vi "testSensorIdToName.vi"(8 "error in (no error)":errorcluster) -> (0 "error out":errorcluster)   [LabVIEW 2016]
doc: "Test the to map the sensor Id to sensor abbreviated name."
uses:
  <vilib>/addons/_JKI Toolkits/Caraya/classes/Test/Test.lvclass
  MatOper/MatOper.lvclass
  <vilib>/addons/_JKI Toolkits/Caraya/classes/Assert/Assert.lvclass
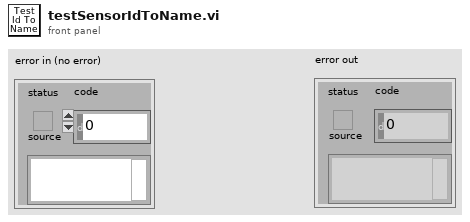
[diagram p1: front panel]
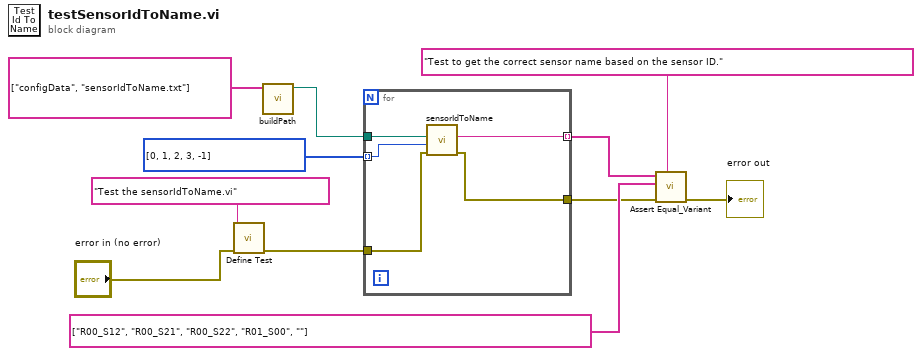
[diagram p0: block diagram]
diagram:
  n1 = call <vilib>:"Define Test.vi"("error in (no error)"="error in (no error)", "Label (VI Title)"="Test the sensorIdToName.vi") -> ("error out"=w8:errorcluster)  [unwired: 9 in]
  n2 = call "buildPath.vi"("Path Name List"=string[] ["configData", "sensorIdToName.txt"]) -> ("New Path"=w1:path)  [unwired: 10 in]
  n3 = for {
    tunnel: i32[] [0, 1, 2, 3, -1] -> [w15] mode=indexing
    tunnel: w1 -> [w16]
    tunnel: w8 -> [w14]
    tunnel: [w13] -> w7 mode=indexing
    tunnel: [w12] -> w5
    n4 = call "sensorIdToName.vi"("error in (no error)"=w14, "Sensor ID"=w15, "Path"=w16) -> ("error out"=w12:errorcluster, "Sensor Name"=w13:string)  [unwired: 6 in, 1 out]
  }
  n5 = call <vilib>:"Assert Equal_Variant.vi"("Label"="Test to get the correct sensor name based on the sensor ID." ("Label (VI Title)"), "error in (no error)"=w5, "Y"=string[] ["R00_S12", "R00_S21", "R00_S22", "R01_S00", ""], "X"=w7) -> ("error out"=→"error out":errorcluster)  [unwired: 7 in]
